vi "PreviousPage.vi"(8 "error in (no error)":errorcluster, 11 "DataBase in":refnum<class "DataBase.lvclass">) -> (0 "error out":errorcluster, 3 "DataBase out":refnum<class "DataBase.lvclass">)   [LabVIEW 2019, in "DataBase.lvlib" / "DataBase.lvclass"]
uses:
  DataBase.lvclass
  DataBase.lvclass/DataBase.ctl
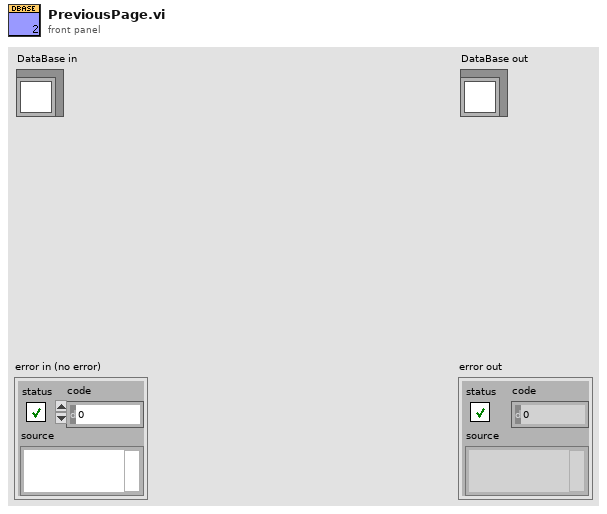
[diagram p1: front panel]
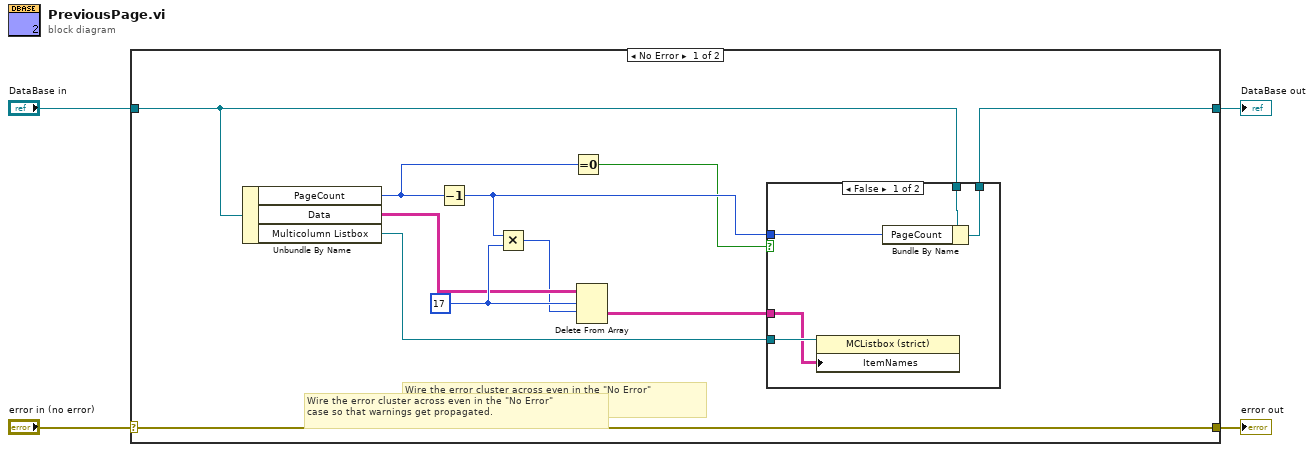
[diagram p0: block diagram]
diagram:
  n1 = case shown="No Error" "error in (no error)" {
    selector: "error in (no error)" -> [w15 w23]
    tunnel: [w15 w23] -> w3
    tunnel: [w5 w22] -> w1
    tunnel: "DataBase in" -> [w6 w22]
    frame No Error {
      w14 = 17 ("length")
      # "Wire the error cluster across even in the \"No Error\"\ncase so that warnings get propagated."
      # "Wire the error cluster across even in the \"No Error\"\ncase so that warnings get propagated."
      n2 = Unbundle By Name(w6) -> ("PageCount"=w8:i32, "Data"=w11:string[][], "Multicolumn Listbox"=w13:refnum<vi>)
      n3 = Decrement(x=w8) -> (x-1=w9:i32)
      n4 = Multiply(x=w9, y=w14) -> (x*y=w10:i32)
      n5 = Equal To 0?(x=w8) -> (x = 0?=w7:bool)
      n6 = Delete From Array(array=w11, length=w14, index (row)=w10) -> (deleted portion=w12:string[][])  [unwired: 1 in, 1 out]
      n7 = case shown="False" w7 {
        tunnel: w13 -> [w20 _]
        tunnel: w12 -> [w19 _]
        tunnel: w6 -> [w18 w21]
        tunnel: w9 -> [w17 _]
        tunnel: [w16 w21] -> w5
        frame False {
          n8 = property class="MCListbox (strict)"(reference=w20, "ItemNames"=w19) -> ()  [unwired: 1 in, 2 out]
          n9 = Bundle By Name(cluster=w18, "PageCount"=w17) -> (w16:refnum<class "DataBase.lvclass">)
        }
        frame True {
        }
      }
    }
    frame Error {
    }
  }
  "error out" <- w3
  "DataBase out" <- w1
